vi "Write.vi"(8 "error in (no error)":errorcluster, 10 "Write Data":variant, 11 "Base Hardware in":refnum<class "Base Hardware.lvclass">) -> (0 "error out":errorcluster, 3 "Base Hardware out":refnum<class "Base Hardware.lvclass">)   [LabVIEW 2023, in "Abstract Hardware.lvlib" / "Base Hardware.lvclass"]
uses:
  Base Hardware.lvclass
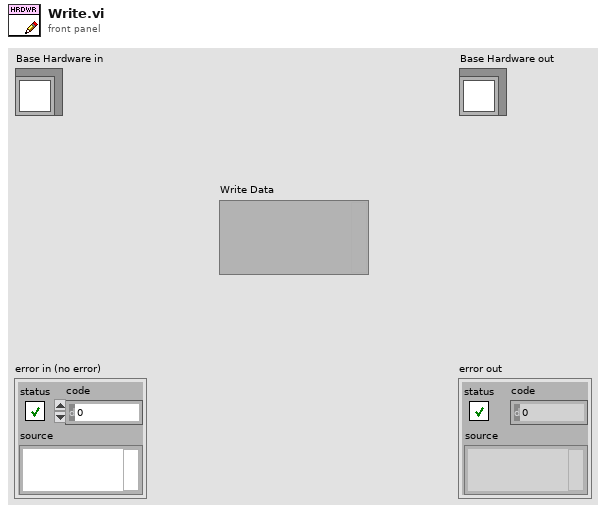
[diagram p1: front panel]
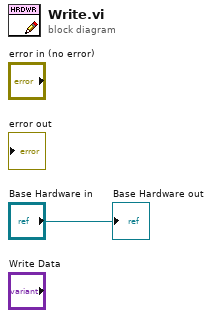
[diagram p0: block diagram]
diagram:
  "Base Hardware out" <- "Base Hardware in"
